vi "Send and log instructions.vi"(5 "prefix":string, 6 "current code":string, 7 "enabled codes":string, 8 "error in (no error)":errorcluster, 10 "instructions":string[](array[string]), 11 "Motor in":refnum<class "Motor.lvclass">) -> (0 "error out":errorcluster, 1 "error":bool, 2 "replies":string[](array[string]), 3 "Motor out":refnum<class "Motor.lvclass">, 4 "ok":bool)   [LabVIEW 2018, in "Motor.lvclass"]
uses:
  Motor.lvclass
  Motor.lvclass/Motor.ctl
panel:
  out "current time 2":timestamp format="%<%H:%M:%S%3u\n%Y/%m/%d>T"
  out "current time":timestamp format="%<%H:%M:%S%3u\n%Y/%m/%d>T"
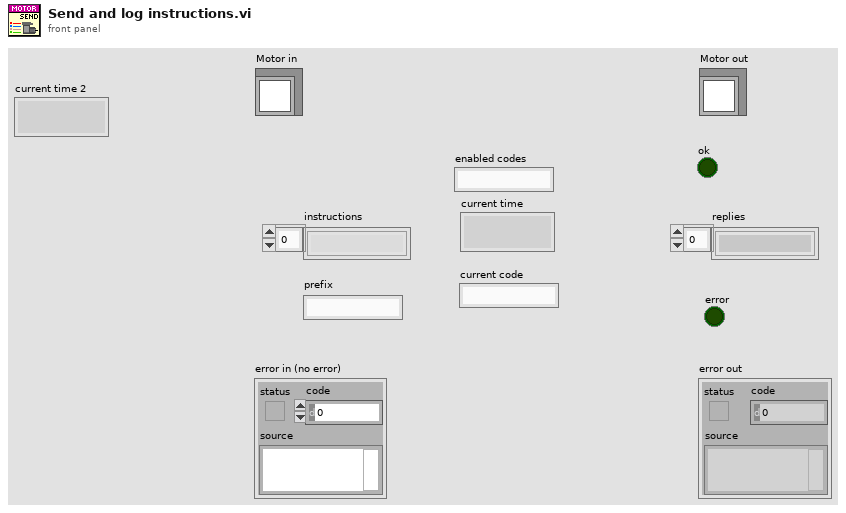
[diagram p1: front panel]
types:
  T1 = enum16{"Standard", "Buffered", "CRLF", "Immediate"}
  T2 = enum16{"open", "replace", "create", "open or create", "replace or create", "replace or create with confirmation"}
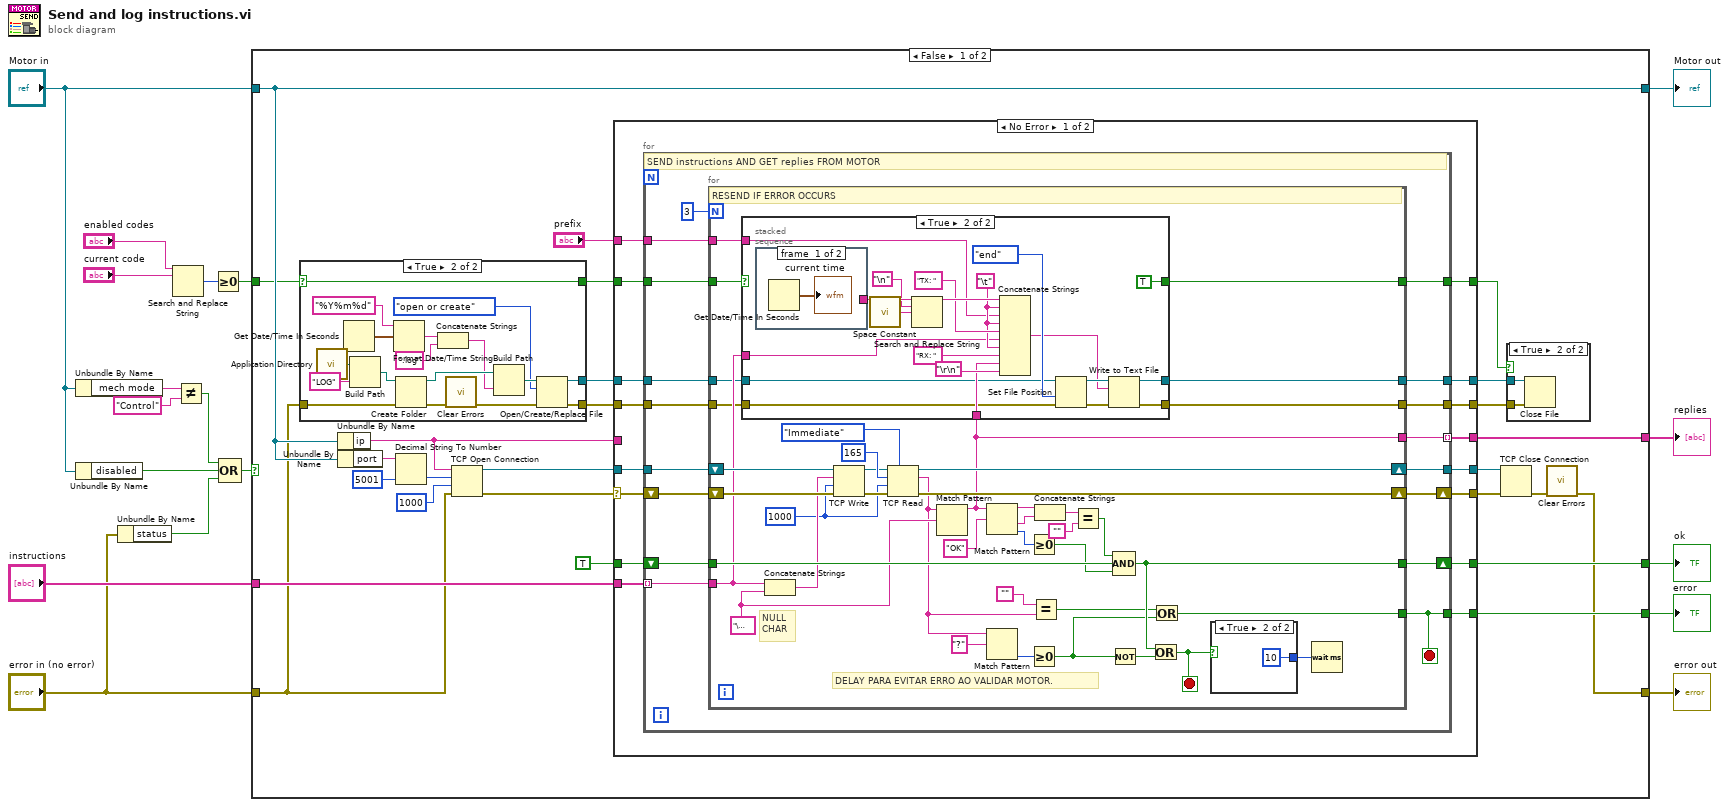
[diagram p0: block diagram]
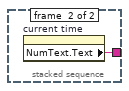
[diagram p3: hidden frame]
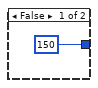
[diagram p4: hidden frame]
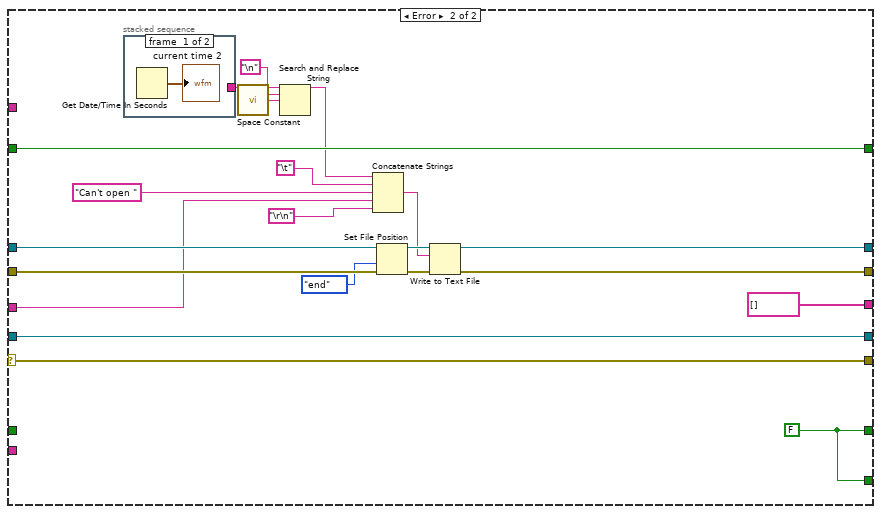
[diagram p5: hidden frame]
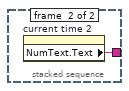
[diagram p6: hidden frame]
diagram:
  n1 = Unbundle By Name("Motor in") -> ("mech mode"=w11:string)
  n2 = Unbundle By Name("Motor in") -> ("disabled"=w8:bool)
  n3 = Unbundle By Name("error in (no error)") -> ("status"=w9:bool)
  n4 = Search and Replace String(input string="enabled codes", search string="current code") -> (number of replacements=w2:i32)  [unwired: 6 in, 3 out]
  n5 = Not Equal?(x=w11, y="Control") -> (x != y?=w5:bool)
  n6 = Greater Or Equal To 0?(x=w2) -> (x >= 0?=w1:bool)
  n7 = Compound Arithmetic op=OR(w5, w8, w9) -> (w7:bool)
  n8 = case shown="False" w7 {
    tunnel: [w30 w189] -> w18
    tunnel: [w44 w190] -> w17
    tunnel: "Motor in" -> [w44 w190]
    tunnel: "instructions" -> [w39 _]
    tunnel: [w37 _] -> w15
    tunnel: [w33 _] -> w14
    tunnel: [w32 _] -> w13
    tunnel: "error in (no error)" -> [w25 w189]
    tunnel: w1 -> [w27 _]
    frame False {
      n9 = case shown="True" w27 {
        selector: w27 -> [w171 w173]
        tunnel: [w170 w175] -> w24
        tunnel: [_ w174] -> w29
        tunnel: [w171 w173] -> w26
        tunnel: w25 -> [w170 w172]
        frame False {
        }
        frame True {
          n10 = call <vilib>:"Application Directory.vi"() -> ("Application Directory"=w180:path)
          n11 = Get Date/Time In Seconds() -> (seconds since 1Jan1904=w181:timestamp)
          n12 = Build Path(base path=w180, name or relative path="LOG") -> (appended path=w185:path)
          n13 = Format Date/Time String(time format string (%c)="%Y%m%d", seconds (now)=w181) -> (date/time string=w182:string)  [unwired: 1 in]
          n14 = Create Folder(path (use dialog)=w185, error in=w172) -> (created path=w188:path, error out=w186:errorcluster)  [unwired: 1 in, 1 out]
          n15 = Concatenate Strings(w182, ".log" ("string")) -> (w184:string)
          n16 = call <vilib>:"Clear Errors.vi"("error in (no error)"=w186) -> ("error out"=w187:errorcluster)  [unwired: 5 in, 1 out]
          n17 = Build Path(base path=w188, name or relative path=w184) -> (appended path=w183:path)
          n18 = Open/Create/Replace File(file path (use dialog)=w183, error in=w187, operation (0:open)=T2."open or create") -> (refnum out=w174:refnum<file>, error out=w175:errorcluster)  [unwired: 3 in, 1 out]
        }
      }
      n19 = Unbundle By Name(w44) -> ("ip"=w19:string)
      n20 = Unbundle By Name(w44) -> ("port"=w42:string)
      n21 = Decimal String To Number(string=w42, default (0L)=u16 5001 ("default (0 I32)")) -> (number=w40:u16)  [unwired: 1 in, 1 out]
      n22 = TCP Open Connection(address=w19, remote port or service name=w40, timeout ms (60000)=1000, error in (no error)=w25) -> (connection ID=w38:refnum<k5>, error out=w20:errorcluster)  [unwired: 1 in]
      n23 = case shown="No Error" w20 {
        selector: w20 -> [w45 w163]
        tunnel: w39 -> [w60 _]
        tunnel: w38 -> [w59 w164]
        tunnel: [w58 w161] -> w37
        tunnel: TRUE -> [w57 _]
        tunnel: [w56 w164] -> w35
        tunnel: [w55 w163] -> w34
        tunnel: [w54 w161] -> w33
        tunnel: [w53 string[] []] -> w32
        tunnel: w29 -> [w52 w156]
        tunnel: "prefix" -> [w51 _]
        tunnel: w26 -> [w50 w165]
        tunnel: w24 -> [w49 w159]
        tunnel: [w48 w157] -> w23
        tunnel: [w47 w155] -> w22
        tunnel: [w46 w165] -> w21
        tunnel: w19 -> [_ w148]
        frame No Error {
          n24 = for {
            tunnel: w60 -> [w77] mode=indexing
            tunnel: w59 -> [w75]
            tunnel: [w70] -> w58
            shift-right: [w74] -> w54
            shift-left: w57 -> [w69]
            tunnel: [w73] -> w56
            shift-right: [w71] -> w55
            shift-left: w45 -> [w76]
            tunnel: [w72] -> w53 mode=indexing
            tunnel: w52 -> [w67]
            tunnel: w51 -> [w66]
            tunnel: w50 -> [w65]
            tunnel: w49 -> [w64]
            tunnel: [w63] -> w48
            tunnel: [w62] -> w47
            tunnel: [w61] -> w46
            stop <- w70 stop-if-true
            # "SEND instructions AND GET replies FROM MOTOR"
            n25 = for {
              N: 3 -> [_]
              tunnel: w77 -> [w86]
              tunnel: [w87] -> w72
              tunnel: [w93] -> w70
              shift-right: [w114] -> w71
              shift-left: w76 -> [w117]
              shift-right: [w115] -> w73
              shift-left: w75 -> [w116]
              tunnel: w69 -> [w113]
              tunnel: [w95] -> w74
              tunnel: w67 -> [w84]
              tunnel: w66 -> [w88]
              tunnel: w65 -> [w85]
              tunnel: w64 -> [w83]
              tunnel: [w82] -> w63
              tunnel: [w81] -> w62
              tunnel: [w80] -> w61
              stop <- w89 stop-if-true
              w107 = 1000 ("timeout ms (60000)")
              w99 = "\u0000" ("search string")
              # "DELAY PARA EVITAR ERRO AO VALIDAR MOTOR."
              # "NULL\nCHAR"
              # "RESEND IF ERROR OCCURS"
              n26 = Concatenate Strings(w86, w99) -> (w108:string)
              n27 = TCP Write(connection ID=w116, data in=w108, error in (no error)=w117, 9:w107) -> (connection ID out=w110:refnum<k5>, error out=w112:errorcluster)  [unwired: 1 out]
              n28 = TCP Read(connection ID=w110, bytes to read=165, error in (no error)=w112, 7:T1."Immediate" ("mode (standard)"), 9:w107) -> (connection ID out=w115:refnum<k5>, data out=w91:string, error out=w114:errorcluster)
              n29 = Match Pattern(string=w91, regular expression=w99) -> (before substring=w87:string)  [unwired: 1 in, 3 out]
              n30 = case shown="True" w85 {
                selector: w85 -> [w118 _]
                tunnel: w88 -> [_ w132]
                tunnel: w87 -> [_ w131]
                tunnel: w86 -> [_ w130]
                tunnel: w84 -> [w120 w128]
                tunnel: w83 -> [w119 w127]
                tunnel: [w119 w124] -> w82
                tunnel: [w120 w123] -> w81
                tunnel: [w118 TRUE] -> w80
                frame False {
                }
                frame True {
                  w135 = "\t"
                  n31 = stacked-sequence {
                    tunnel: [_ w142] -> w140
                    frame #0 {
                      n32 = Get Date/Time In Seconds() -> (seconds since 1Jan1904=→"current time":timestamp)
                    }
                    frame #1 {
                      n33 = property on="current time" class="AbsTime (strict)"() -> ("NumText.Text"=w142:string)  [unwired: 2 in, 2 out]
                    }
                  }
                  n34 = call <vilib>:"Space Constant.vi"() -> ("String"=w138:string)
                  n35 = Search and Replace String(input string=w140, search string="\n", replace string=w138) -> (result string=w137:string)  [unwired: 5 in, 3 out]
                  n36 = Concatenate Strings(w137, w135, w132, w135, "TX: ", w130, w135, "RX: ", w131, "\r\n") -> (w122:string)
                  n37 = Set File Position(refnum=w128, from (0:start)=enum16{"start", "end", "current"}."end", error in=w127) -> (refnum out=w125:refnum<file>, error out=w126:errorcluster)  [unwired: 1 in]
                  n38 = Write to Text File(file (use dialog)=w125, text=w122, error in=w126) -> (refnum out=w123:refnum<file>, error out=w124:errorcluster)  [unwired: 1 in, 1 out]
                }
              }
              n39 = Match Pattern(string=w87, regular expression="OK" ("y")) -> (before substring=w101:string, after substring=w104:string, offset past match=w98:i32)  [unwired: 1 in, 1 out]
              n40 = Match Pattern(string=w91, regular expression="?") -> (offset past match=w106:i32)  [unwired: 1 in, 3 out]
              n41 = Greater Or Equal To 0?(x=w98) -> (x >= 0?=w96:bool)
              n42 = Greater Or Equal To 0?(x=w106) -> (x >= 0?=w94:bool)
              n43 = Equal?(x="", y=w91) -> (x = y?=w92:bool)
              n44 = Concatenate Strings(w101, w104) -> (w102:string)
              n45 = Equal?(x=w102, y="") -> (x = y?=w97:bool)
              n46 = Not(x=w94) -> (.not. x?=w79:bool)
              n47 = Compound Arithmetic op=AND(w97, w113, w96) -> (w95:bool)
              n48 = Or(x=w95, y=w79) -> (x .or. y?=w89:bool)
              n49 = Or(x=w92, y=w94) -> (x .or. y?=w93:bool)
              n50 = case shown="True" w89 {
                tunnel: [u32 150 ("milliseconds to wait") u32 10 ("milliseconds to wait")] -> w78
                frame False {
                }
                frame True {
                }
              }
              n51 = Wait (ms)(milliseconds to wait=w78) -> ()  [unwired: 1 out]
            }
          }
        }
        frame Error {
          w161 = FALSE
          n52 = stacked-sequence {
            tunnel: [_ w167] -> w152
            frame #0 {
              n53 = Get Date/Time In Seconds() -> (seconds since 1Jan1904=→"current time 2":timestamp)
            }
            frame #1 {
              n54 = property on="current time 2" class="AbsTime (strict)"() -> ("NumText.Text"=w167:string)  [unwired: 2 in, 2 out]
            }
          }
          n55 = call <vilib>:"Space Constant.vi"() -> ("String"=w151:string)
          n56 = Search and Replace String(input string=w152, search string="\n", replace string=w151) -> (result string=w146:string)  [unwired: 5 in, 3 out]
          n57 = Concatenate Strings(w146, "\t", "Can't open " ("string"), w148, "\r\n") -> (w154:string)
          n58 = Set File Position(refnum=w156, from (0:start)=enum16{"start", "end", "current"}."end", error in=w159) -> (refnum out=w160:refnum<file>, error out=w158:errorcluster)  [unwired: 1 in]
          n59 = Write to Text File(file (use dialog)=w160, text=w154, error in=w158) -> (refnum out=w155:refnum<file>, error out=w157:errorcluster)  [unwired: 1 in, 1 out]
        }
      }
      n60 = TCP Close Connection(connection ID=w35, error in (no error)=w34) -> (error out=w31:errorcluster)  [unwired: 1 in, 1 out]
      n61 = case shown="True" w21 {
        tunnel: w23 -> [_ w169]
        tunnel: w22 -> [_ w168]
        frame False {
        }
        frame True {
          n62 = Close File(refnum=w168, error in=w169) -> ()  [unwired: 2 out]
        }
      }
      n63 = call <vilib>:"Clear Errors.vi"("error in (no error)"=w31) -> ("error out"=w30:errorcluster)  [unwired: 5 in, 1 out]
    }
    frame True {
    }
  }
  "error out" <- w18
  "Motor out" <- w17
  "error" <- w15
  "ok" <- w14
  "replies" <- w13
